vi "test_gen_noisy_array.vi"() -> ()   [LabVIEW 2022 SP3]
uses:
  <vilib>/Analysis/baseanly.llb/Mean (DBL).vi
  <vilib>/Analysis/NI_AALBase.lvlib
panel:
  out "mean":dbl format="%0.4f"
  in  "Stop Button":bool
  in  "Slider":dbl(slide) scale=0.0..10.0
  out "Intensity Graph":dbl[][](graph)
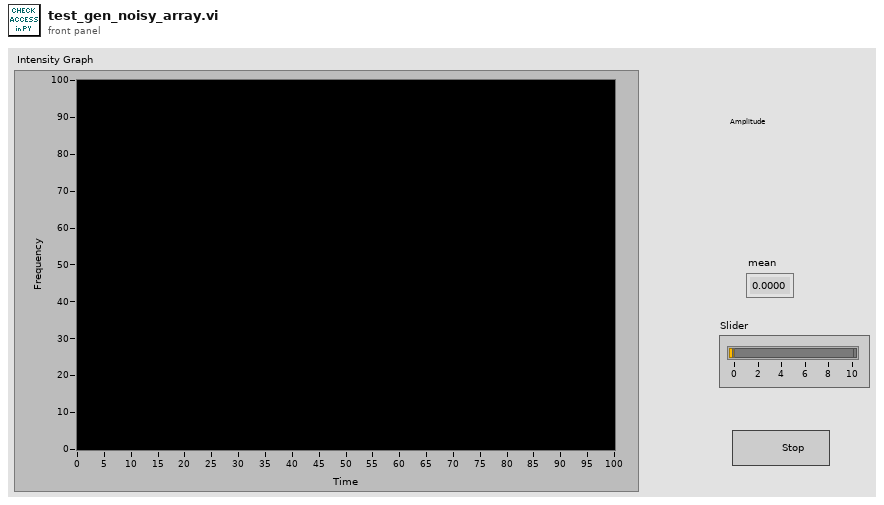
[diagram p1: front panel]
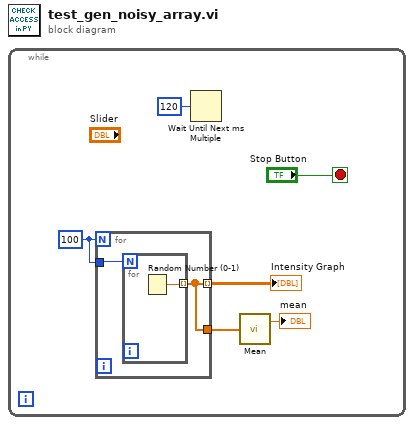
[diagram p0: block diagram]
diagram:
  n1 = while {
    stop <- "Stop Button" stop-if-true
    w5 = 100
    n2 = for {
      N: w5 -> [_]
      tunnel: [w7] -> w4 mode=indexing
      tunnel: w5 -> [w8]
      tunnel: [w7] -> w3
      n3 = for {
        N: w8 -> [_]
        tunnel: [w9] -> w7 mode=indexing
        n4 = Random Number (0-1)() -> (number: 0 to 1=w9:dbl)
      }
    }
    "Intensity Graph" <- w4
    n5 = Wait Until Next ms Multiple(millisecond multiple=u32 120) -> ()  [unwired: 1 out]
    n6 = call-poly <vilib>:"Mean.vi"("X"=w3) -> ("mean"=→"mean":dbl)  [unwired: 1 out]
  }
